vi "main_80MHz.vi"() -> ()   [LabVIEW 2010]
uses:
  common_typedefs/channels_cluster.ctl
  common_typedefs/gate_parameters_cluster.ctl
  <vilib>/Platform/TimedLoop/XDataNode/XDataNode.xnode
  <vilib>/Platform/TimedLoop/XDataNode/timing_clust.ctl
  <vilib>/Platform/TimedLoop/XDataNode/nitl_modes.ctl
  <vilib>/Platform/TimedLoop/XDataNode/wakeup.ctl
  <vilib>/eio/EIONode/EIONode.xnode
  <vilib>/rvi/eio/nirviEIOImplementation/nirviEIOImplementation.xnode
  <vilib>/rvi/eio/common/nirviEmuClasses.ctl
  <vilib>/rvi/eio/common/nirviEmuTemplateMethod_noerrors.vi
  <vilib>/Platform/TimedLoop/XDataNode/XDNodeRunTimeDep.lvlib
panel:
  out "Input0":bool
  out "Input1":bool
  out "clamp first pixel? 2":bool
  in  "clamp first pixel?":bool
  in  "gate 3":T1
  in  "gate 2":T1
  in  "gate 1":T1
  out "integrated pixel values":T2
  out "data read":T2
  out "clock 3 state":bool
  out "clock 2 state":bool
  out "clock 1 state":bool
  in  "stop acquisition at FIFO overflow?":bool=TRUE
  in  "wait for trigger?":bool
  in  "stop":bool
  in  "acquire":bool
  out "acquiring?":bool
  out "FIFO overflow":bool
  out "current pixel no.":i64
  in  "number of pixels":i64=-1
  in  "maximum bit depth":i8
  in  "iterations per pixel":u32
  in  "enable ADC clock?":bool=TRUE
  in  "ADC clock phase":u8
  # "Outputs / displays"
  # "Integration parameters"
  # "Clock parameters"
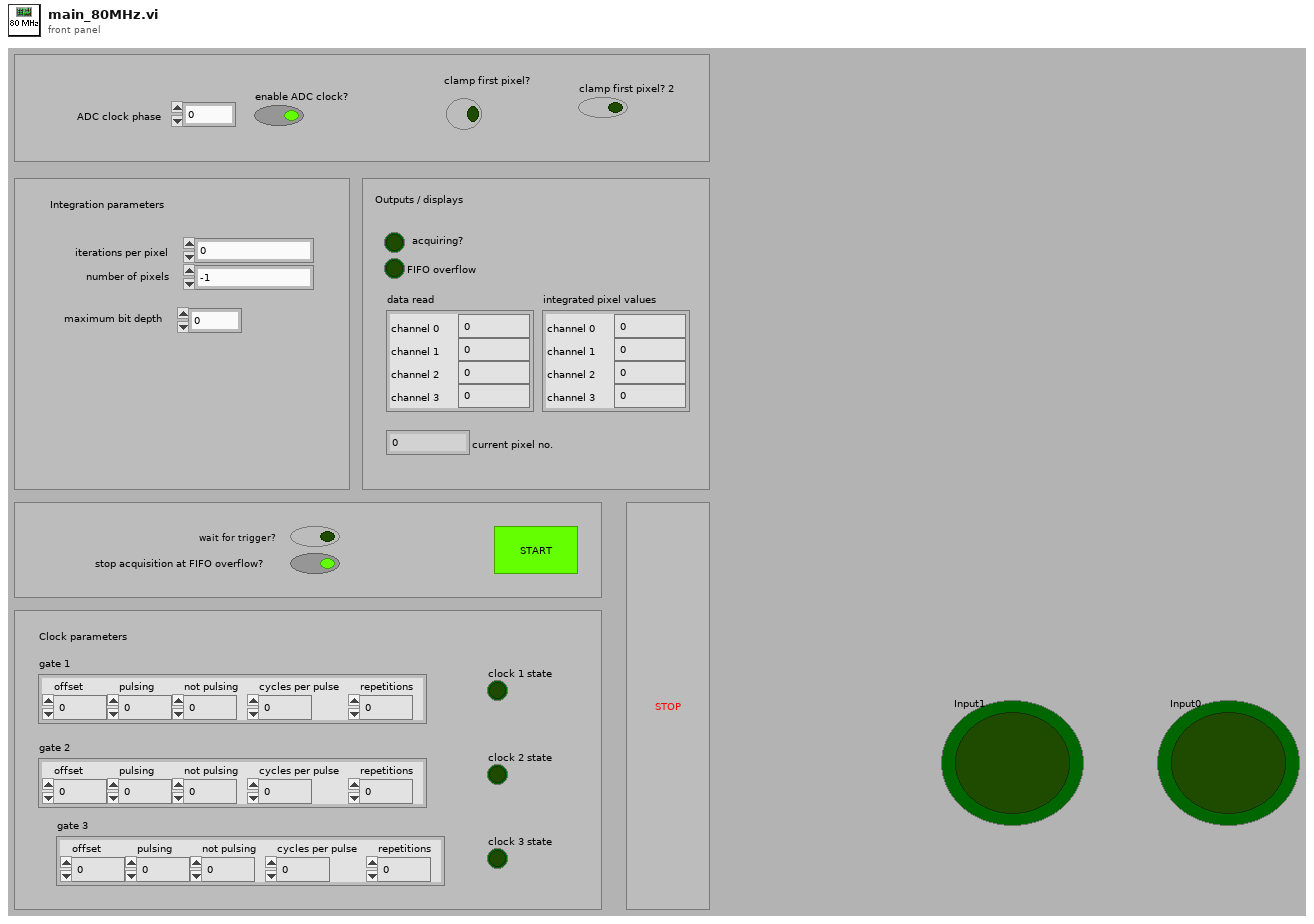
[diagram p1: front panel]
types:
  T1 = typedef "gate_parameters_cluster.ctl" = cluster{"offset":i64, "pulsing":i64, "not pulsing":i64, "cycles per pulse":i64, "repetitions":i64}
  T2 = typedef "channels_cluster.ctl" = cluster{"channel 0":u32, "channel 1":u32, "channel 2":u32, "channel 3":u32}
  T3 = typedef "XDNodeRunTimeDep.lvlib/timing_clust.ctl" = cluster{"Expected End [f-1]":u64, "Actual End [f-1]":u64, "Finished Late? [f-1]":bool, "Expected End [i-1]":u64, "Actual End [i-1]":u64, "Finished Late? [i-1]":bool, "Expected Start [i]":u64, "Actual Start [i]":u64, "Expected Start [f]":u64, "Actual Start [f]":u64, "Source Name":string, "Structure Name":string, "Period":i64, "Deadline":i64, "Offset":i64, "Start":i64, "Priority":i32, "Timeout":i32, "Mode":T4, "Wakeup Reason":T5, "Error":errorcluster, "Source Type":string, "Secondary Source Type":string, "Global End Time":u64, "Global Start Time":u64, "Frame Duration":u64, "Iteration Duration":u64, "Assigned CPU":i32, "I/O Scan Engine Mode":u32}
  T4 = typedef "XDNodeRunTimeDep.lvlib/nitl_modes.ctl" = enum32{"No Change", "Process missed periods, maintain original phase", "Discard missed periods, maintain original phase", "Process missed periods, ignore original phase", "Discard missed periods, ignore original phase"}
  T5 = typedef "XDNodeRunTimeDep.lvlib/wakeup.ctl" = enum32{"Normal", "Aborted", "Asynchronous wakeup", "Timing source error", "Timed loop error", "Timeout"}
  T6 = typedef "nirviEmuClasses.ctl" = enum16{"IO Read", "IO Write", "Method", "Property Read", "Property Write"}
  T7 = typedef "gate_counters_cluster.ctl" = cluster{"phase iteration counter":i64, "phase repetition counter":i64, "pulse iteration counter":i64, "phase state":bool}
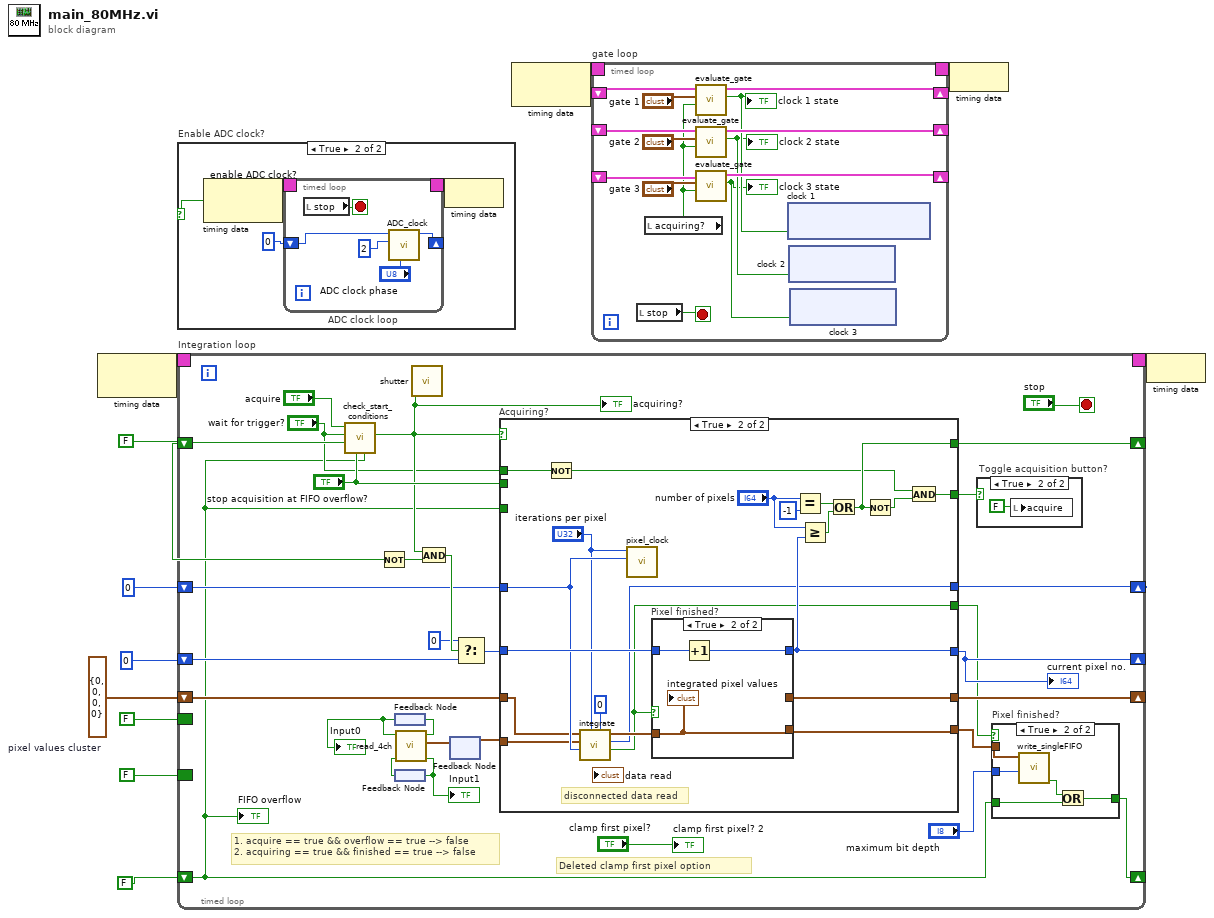
[diagram p0: block diagram]
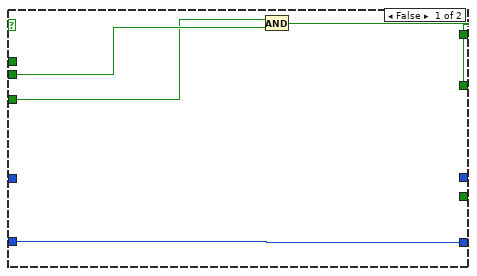
[diagram p4: hidden frame]
diagram:
  w6 = T2 {"channel 0"=0, "channel 1"=0, "channel 2"=0, "channel 3"=0}  # pixel values cluster
  n1 = node-c288() -> (w11:T3)  [unwired: 1 in]
  n2 = case "Enable ADC clock?" shown="True" "enable ADC clock?" {
    frame False {
    }
    frame True {
      n3 = node-c288() -> (w15:T3)  [unwired: 1 in]
      n4 = timed-loop "ADC clock loop" {
        timing: w15 -> [_]
        timing-out: [_] -> w14
        shift-right: [w19] -> _
        shift-left: u8 0 ("counter out") -> [w20]
        stop <- w17 stop-if-true
        n5 = local read "stop"() -> (w17:bool)
        n6 = call "ADC_clock.vi"("phase"="ADC clock phase", "iterations per cycle"=u8 2, "counter in"=w20) -> ("counter out"=w19:u8)  [unwired: 8 in]
      }
      n7 = node-c288(w14) -> ()
    }
  }
  n8 = timed-loop "Integration loop" {
    timing: w11 -> [_]
    timing-out: [_] -> w10
    shift-right: [w36] -> _
    shift-left: i64 0 -> [w39]
    shift-right: [w51] -> _
    shift-left: u32 0 ("iteration counter out") -> [w35]
    shift-right: [w52] -> _
    shift-left: w6 -> [w53]
    shift-right: [w45] -> _
    shift-left: FALSE -> [w25]
    shift-right: [w47] -> _
    shift-left: FALSE -> [w33]
    border: FALSE ("Connector1/DIO0") -> [_]
    border: FALSE ("Connector1/DIO1") -> [_]
    stop <- "stop" stop-if-true
    # "Deleted clamp first pixel option"
    # "1. acquire == true && overflow == true --> false\n2. acquiring == true && finished == true --> false"
    n9 = call "check_start_conditions.vi"("FIFO overflow?"=w25, "stop at FIFO overflow?"="stop acquisition at FIFO overflow?", "already acquiring?"=w33, "in triggered mode?"="wait for trigger?", "acquire"="acquire") -> ("acquire?"=w42:bool)  [unwired: 6 in]
    "acquiring?" <- w42
    n10 = Not(x=w33) -> (.not. x?=w41:bool)
    n11 = feedback #1() -> (w29:bool)
    "Input0" <- w29
    n12 = feedback #2() -> (w31:bool)
    n13 = call "read_4ch.vi"("previous value ch1"=w31, "previous value ch0"=w29) -> ("Inputl1"=w30:bool, "read output"=w50:T2, "Input0"=w32:bool)  [unwired: 7 in]
    "Input1" <- w30
    n14 = feedback-in #1(w32) -> ()
    n15 = feedback-in #2(w30) -> ()
    n16 = call "shutter.vi"("open?"=w42) -> ()  [unwired: 11 in]
    n17 = And(x=w42, y=w41) -> (x .and. y?=w40:bool)
    n18 = feedback-in #3(w50) -> ()
    n19 = feedback #3() -> (w49:T2)  [unwired: 1 in]
    n20 = Select(t=i64 0, s=w40, f=w39) -> (s? t:f=w38:i64)
    n21 = case "Acquiring?" shown="True" w42 {
      tunnel: [_ w68] -> w46
      tunnel: [_ w69] -> w51
      tunnel: [w62 w83] -> w36
      tunnel: w53 -> [_ w77]
      tunnel: w38 -> [w62 w81]
      tunnel: w35 -> [_ w79]
      tunnel: [_ w82] -> w52
      tunnel: w49 -> [_ w78]
      tunnel: "stop acquisition at FIFO overflow?" -> [w65 _]
      tunnel: [_ w73] -> w47
      tunnel: [w63 w71] -> w44
      tunnel: w25 -> [w64 _]
      tunnel: "wait for trigger?" -> [_ w72]
      tunnel: [_ w70] -> w34
      frame False {
        n22 = And(x=w64, y=w65) -> (x .and. y?=w63:bool)
      }
      frame True {
        # "disconnected data read"
        n23 = Not(x=w72) -> (.not. x?=w67:bool)
        n24 = call "integrate.vi"("waiting iterations per pixel"=u32 0, "integration iterations per pixel"="iterations per pixel", "iteration counter in"=w79, "sampling values in"=w78, "previous pixel values in"=w77) -> ("finished?"=w70:bool, "iteration counter out"=w69:u32, "new pixel values out"=w80:T2)  [unwired: 4 in]
        n25 = call "pixel_clock.vi"("current iteration"=w79, "iterations per pixel"="iterations per pixel") -> ()  [unwired: 10 in]
        n26 = case "Pixel finished?" shown="True" w70 {
          tunnel: w80 -> [w87 w89]
          tunnel: [_ w89] -> w68
          tunnel: [w88 w90] -> w83
          tunnel: w81 -> [w88 w91]
          tunnel: [w87 _] -> w82
          frame False {
          }
          frame True {
            n27 = Increment(x=w91) -> (x+1=w90:i64)
            "integrated pixel values" <- w89
          }
        }
        n28 = Equal?(x="number of pixels", y=i64 -1 ("x")) -> (x = y?=w86:bool)
        n29 = Greater Or Equal?(x="number of pixels", y=w83) -> (x >= y?=w85:bool)
        n30 = Or(x=w86, y=w85) -> (x .or. y?=w73:bool)
        n31 = Not(x=w73) -> (.not. x?=w66:bool)
        n32 = And(x=w67, y=w66) -> (x .and. y?=w71:bool)
      }
    }
    "current pixel no." <- w36
    n33 = case "Toggle acquisition button?" shown="True" w44 {
      frame False {
      }
      frame True {
        n34 = local write "acquire"(FALSE) -> ()
      }
    }
    n35 = case "Pixel finished?" shown="True" w34 {
      tunnel: w46 -> [_ w56]
      tunnel: [w55 w58] -> w45
      tunnel: w25 -> [w55 w57]
      tunnel: "maximum bit depth" -> [_ w60]
      frame False {
      }
      frame True {
        n36 = call "write_singleFIFO.vi"("maximum bit depth"=w60, "values to be written"=w56) -> ("FIFO overflow"=w59:bool)  [unwired: 9 in]
        n37 = Or(x=w59, y=w57) -> (x .or. y?=w58:bool)
      }
    }
    "FIFO overflow" <- w25
    "clamp first pixel? 2" <- "clamp first pixel?"
  }
  n38 = node-c288() -> (w5:T3)  [unwired: 1 in]
  n39 = timed-loop "gate loop" {
    timing: w5 -> [_]
    timing-out: [_] -> w4
    shift-right: [w106] -> _
    shift-left: _ -> [w107]
    shift-right: [w104] -> _
    shift-left: _ -> [w105]
    shift-right: [w103] -> _
    shift-left: _ -> [w102]
    stop <- w97 stop-if-true
    n40 = local read "stop"() -> (w97:bool)
    n41 = local read "acquiring?"() -> (w98:bool)
    n42 = call "evaluate_gate.vi"("acquiring?"=w98, "gate settings"="gate 1", "gate counters in"=w107) -> ("pulse state out"=w96:bool, "gate counters out"=w106:T7)  [unwired: 7 in]
    "clock 1 state" <- w96
    n43 = call "evaluate_gate.vi"("acquiring?"=w98, "gate settings"="gate 2", "gate counters in"=w105) -> ("pulse state out"=w95:bool, "gate counters out"=w104:T7)  [unwired: 7 in]
    "clock 2 state" <- w95
    n44 = call "evaluate_gate.vi"("acquiring?"=w98, "gate settings"="gate 3", "gate counters in"=w102) -> ("pulse state out"=w94:bool, "gate counters out"=w103:T7)  [unwired: 7 in]
    "clock 3 state" <- w94
    n45 = xnode "clock 1"("Connector1/DIO32"=w96) -> ()  [unwired: 1 in, 1 out]
    n46 = xnode "clock 2"("PCIe_RTSI_1"=w95) -> ()  [unwired: 1 in, 1 out]
    n47 = xnode "clock 3"("PCIe_RTSI_2"=w94) -> ()  [unwired: 1 in, 1 out]
  }
  n48 = node-c288(w4) -> ()
  n49 = node-c288(w10) -> ()
